vi "Check Status.vi"(8 "error in (no error)":errorcluster, 11 "Magna Power in":refnum<class "Magna Power.lvclass">) -> (0 "error out":errorcluster, 1 "Status":string, 2 "Ready?":bool, 3 "Magna Power out":refnum<class "Magna Power.lvclass">)   [LabVIEW 2012, in "Magna Power.lvclass"]
doc: "(Dynamic) Check if the instrument is powered on and update its member fields with the instrument's current status. Optionally return a text status message."
uses:
  Magna Power.lvclass
  Magna Power.lvclass/Magna Power.ctl
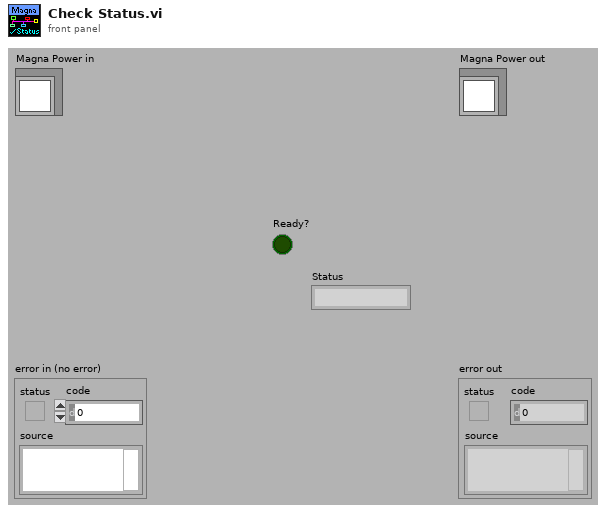
[diagram p1: front panel]
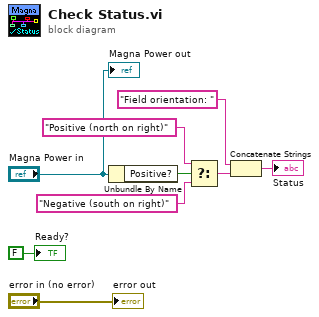
[diagram p0: block diagram]
diagram:
  n1 = Unbundle By Name("Magna Power in") -> ("Positive?"=w4:bool)
  n2 = Select(t="Positive (north on right)", s=w4, f="Negative (south on right)") -> (s? t:f=w3:string)
  n3 = Concatenate Strings("Field orientation: ", w3) -> (→"Status":string)
  "error out" <- "error in (no error)"
  "Magna Power out" <- "Magna Power in"
  "Ready?" <- FALSE ("Ready?")
